vi "ReplaceTags.vi"(10 "Path in":string) -> (2 "Path out":string)   [LabVIEW 2020]
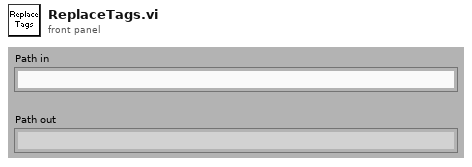
[diagram p1: front panel]
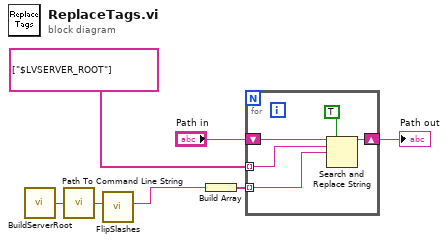
[diagram p0: block diagram]
diagram:
  n1 = call <vilib>:"BuildServerRoot.vi"() -> ("Server Root"=w3:path)
  n2 = call <vilib>:"Path To Command Line String.vi"("path"=w3) -> ("string"=w2:string)
  n3 = call <vilib>:"FlipSlashes.vi"("Before"=w2) -> ("After"=w1:string)  [unwired: 1 in, 9 out]
  n4 = Build Array(w1) -> (w6:string[])
  n5 = for {
    tunnel: w6 -> [w10] mode=indexing
    tunnel: string[] ["$LVSERVER_ROOT"] -> [w11] mode=indexing
    shift-right: [w8] -> w4
    shift-left: "Path in" -> [w12]
    n6 = Search and Replace String(replace all?=TRUE ("replace all? (F)"), input string=w12, search string=w11, replace string=w10) -> (result string=w8:string)  [unwired: 1 in, 6 out]
  }
  "Path out" <- w4
